vi "BuildFindFirstSlotQuery.vi"(8 "error in (no error)":errorcluster, 10 "Array":T1[](array[typedef]), 11 "Table":string) -> (0 "error out":errorcluster, 3 "String":string)   [LabVIEW 2020]
uses:
  DataTypes/SlotPriority--Cluster.ctl
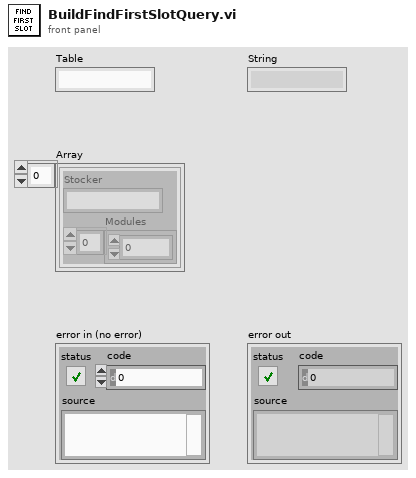
[diagram p1: front panel]
types:
  T1 = typedef "SlotPriority--Cluster.ctl" = cluster{"Stocker":string, "Modules":i32[]}
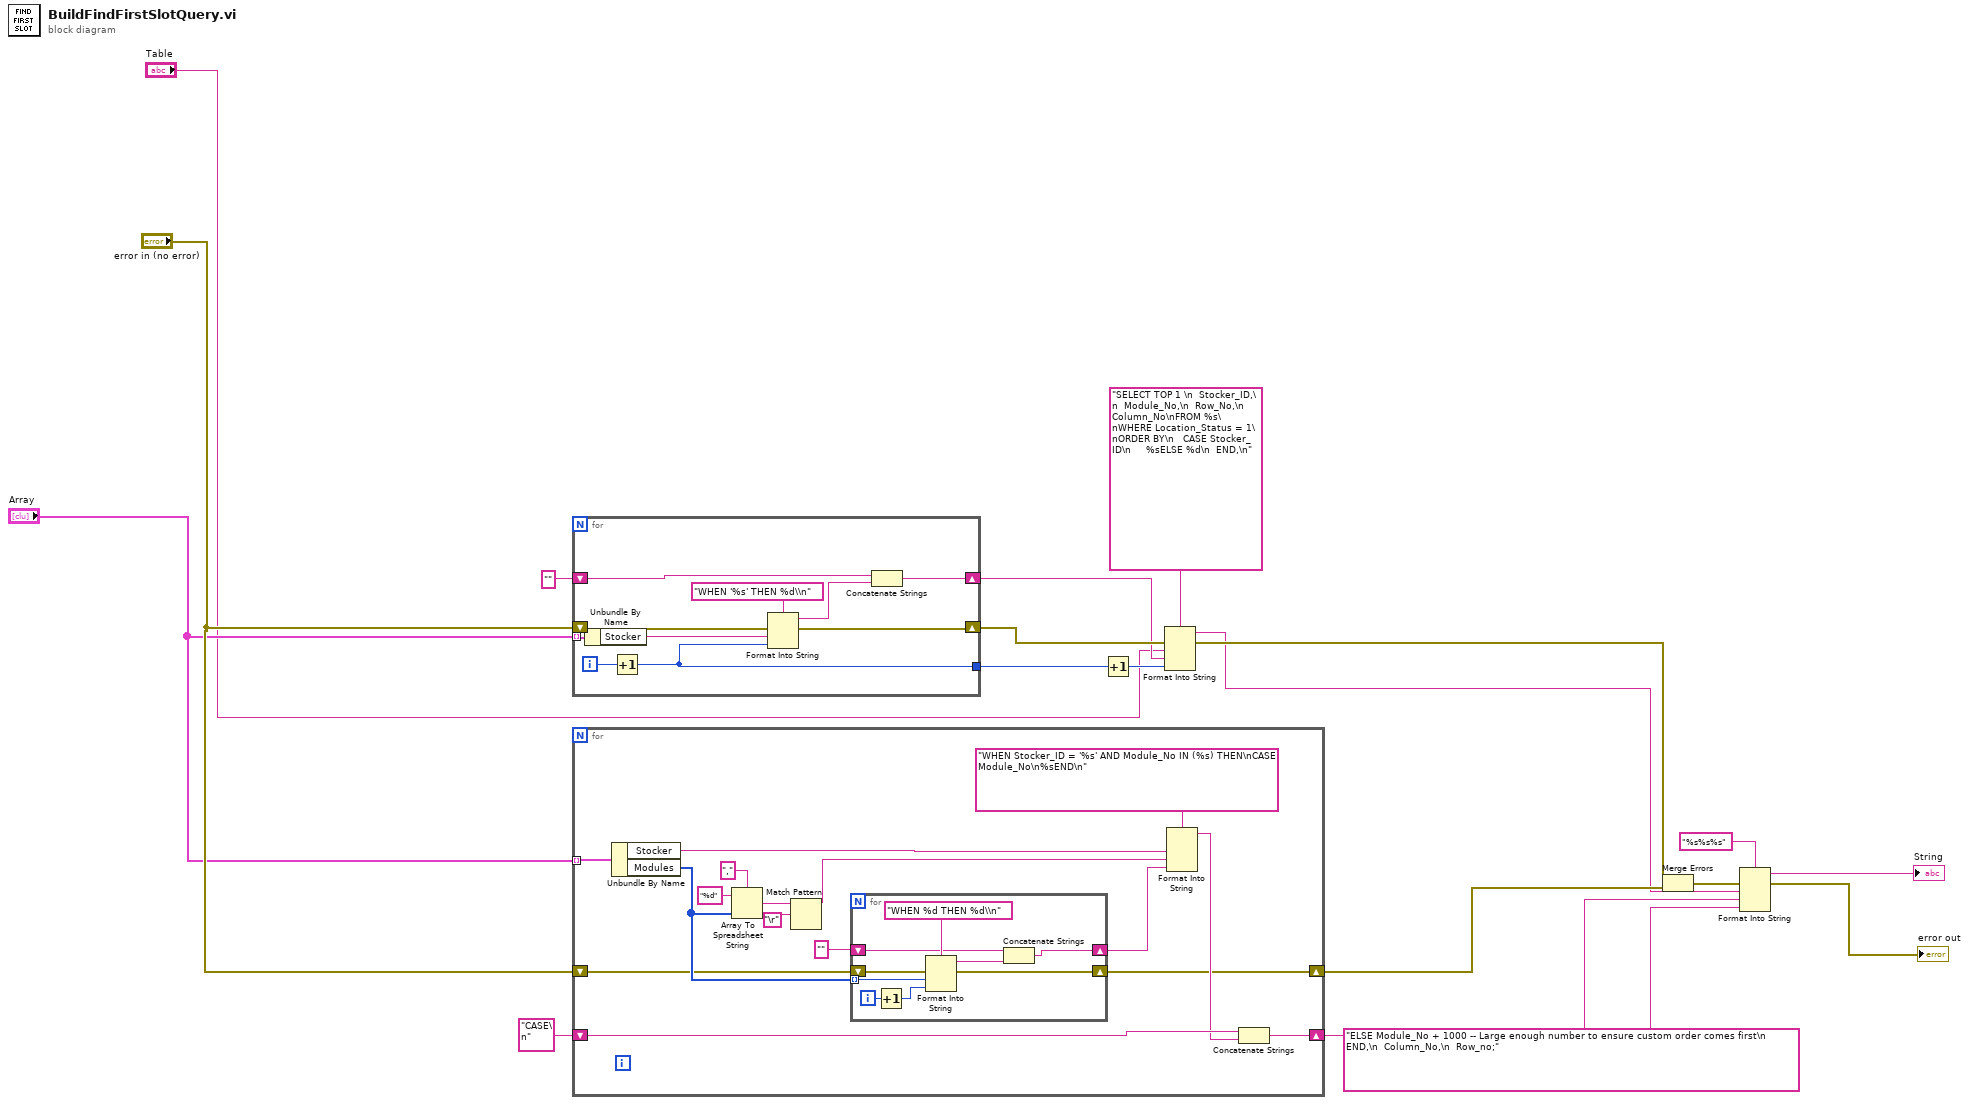
[diagram p0: block diagram]
diagram:
  n1 = for {
    tunnel: "Array" -> [w29] mode=indexing
    shift-right: [w24] -> w5
    shift-left: "" -> [w25]
    tunnel: [w22] -> w2
    shift-right: [w20] -> w17
    shift-left: "error in (no error)" -> [w21]
    i -> [w23]
    n2 = Unbundle By Name(w29) -> ("Stocker"=w27:string)
    n3 = Increment(x=w23) -> (x+1=w22:i32)
    n4 = Format Into String(format string="WHEN '%s' THEN %d\\n", error in=w21, w27, w22) -> (resulting string=w26:string, error out=w20:errorcluster)  [unwired: 1 in]
    n5 = Concatenate Strings(w25, w26) -> (w24:string)
  }
  n6 = for {
    tunnel: "Array" -> [w45] mode=indexing
    shift-right: [w32] -> w11
    shift-left: "CASE\n" -> [w39]
    shift-right: [w30] -> w19
    shift-left: "error in (no error)" -> [w31]
    n7 = Unbundle By Name(w45) -> ("Stocker"=w40:string, "Modules"=w43:i32[])
    n8 = Array To Spreadsheet String(delimiter (Tab)=",", array=w43, 3:"%d" ("format string")) -> (spreadsheet string=w36:string)
    n9 = Match Pattern(string=w36, regular expression="\r") -> (before substring=w35:string)  [unwired: 1 in, 3 out]
    n10 = for {
      tunnel: w43 -> [w53] mode=indexing
      shift-right: [w48] -> w34
      shift-left: "" -> [w51]
      shift-right: [w46] -> w30
      shift-left: w31 -> [w47]
      i -> [w49]
      n11 = Increment(x=w49) -> (x+1=w50:i32)
      n12 = Format Into String(format string="WHEN %d THEN %d\\n", error in=w47, w53, w50) -> (resulting string=w52:string, error out=w46:errorcluster)  [unwired: 1 in]
      n13 = Concatenate Strings(w51, w52) -> (w48:string)
    }
    n14 = Format Into String(format string="WHEN Stocker_ID = '%s' AND Module_No IN (%s) THEN\nCASE Module_No\n%sEND\n", w40, w35, w34) -> (resulting string=w33:string)  [unwired: 2 in, 1 out]
    n15 = Concatenate Strings(w39, w33) -> (w32:string)
  }
  n16 = Increment(x=w2) -> (x+1=w6:i32)
  n17 = Format Into String(format string="SELECT TOP 1 \n  Stocker_ID,\n  Module_No,\n  Row_No,\n  Column_No\nFROM %s\nWHERE Location_Status = 1\nORDER BY\n   CASE Stocker_ID\n     %sELSE %d\n  END,\n", error in=w17, "Table", w5, w6) -> (resulting string=w9:string, error out=w14:errorcluster)  [unwired: 1 in]
  n18 = Merge Errors(w14, w19) -> (w18:errorcluster)
  n19 = Format Into String(format string="%s%s%s", error in=w18, w9, w11, "ELSE Module_No + 1000 -- Large enough number to ensure custom order comes first\n  END,\n  Column_No,\n  Row_no;" ("input 3")) -> (resulting string=→"String":string, error out=→"error out":errorcluster)  [unwired: 1 in]
